vi "Make Necessary Directories.vi"(8 "error in":errorcluster, 11 "Path":path) -> (0 "error out":errorcluster, 3 "Duplicated path":path)   [LabVIEW 2013]
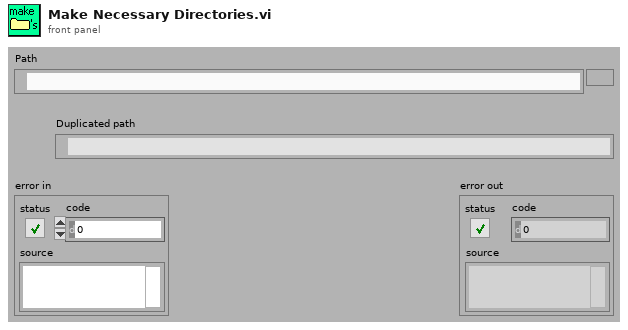
[diagram p1: front panel]
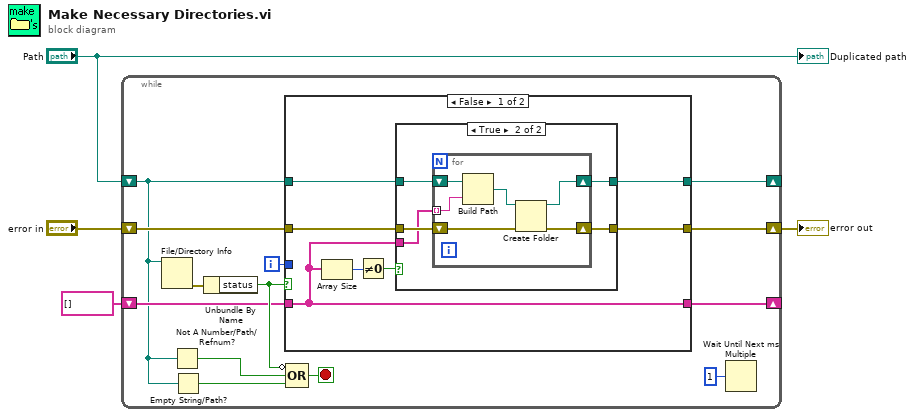
[diagram p0: block diagram]
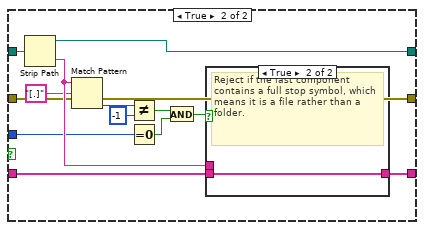
[diagram p3: hidden frame]
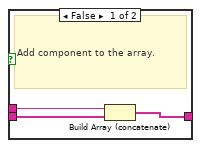
[diagram p4: hidden frame]
diagram:
  n1 = while {
    shift-right: [w14] -> _
    shift-left: "Path" -> [w8]
    shift-right: [w12] -> _
    shift-left: string[] [] -> [w13]
    shift-right: [w9] -> w1
    shift-left: "error in" -> [w10]
    i -> [w5]
    stop <- w16 stop-if-true
    n2 = File/Directory Info(path=w8) -> (error out=w17:errorcluster)  [unwired: 1 in, 6 out]
    n3 = Not A Number/Path/Refnum?(number/path/refnum=w8) -> (NaN/Path/Refnum?=w7:bool)
    n4 = Empty String/Path?(string/path=w8) -> (empty?=w6:bool)
    n5 = Unbundle By Name(w17) -> ("status"=w15:bool)
    n6 = case shown="False" w15 {
      tunnel: w8 -> [w24 w43]
      tunnel: [w23 w50] -> w14
      tunnel: w13 -> [w18 w49]
      tunnel: [w18 w48] -> w12
      tunnel: w10 -> [w22 w42]
      tunnel: [w19 w42] -> w9
      tunnel: w5 -> [_ w39]
      frame False {
        n7 = Array Size(array=w18) -> (size(s)=w20:i32)
        n8 = Not Equal To 0?(x=w20) -> (x != 0?=w21:bool)
        n9 = case shown="True" w21 {
          tunnel: w24 -> [w26 w31]
          tunnel: [w26 w29] -> w23
          tunnel: w22 -> [w25 w28]
          tunnel: w18 -> [_ w27]
          tunnel: [w25 w30] -> w19
          frame False {
          }
          frame True {
            n10 = for {
              shift-right: [w33] -> w29
              shift-left: w31 -> [w37]
              tunnel: w27 -> [w32] mode=indexing
              shift-right: [w34] -> w30
              shift-left: w28 -> [w35]
              n11 = Build Path(base path=w37, name or relative path=w32) -> (appended path=w36:path)
              n12 = Create Folder(path (use dialog)=w36, error in=w35) -> (created path=w33:path, error out=w34:errorcluster)  [unwired: 2 out]
            }
          }
        }
      }
      frame True {
        n13 = Strip Path(path=w43) -> (stripped path=w50:path, name=w47:string)
        n14 = Match Pattern(string=w47, regular expression="[.]") -> (offset past match=w46:i32)  [unwired: 4 out]
        n15 = Not Equal?(x=w46, y=-1) -> (x != y?=w41:bool)
        n16 = Equal To 0?(x=w39) -> (x = 0?=w38:bool)
        n17 = And(x=w41, y=w38) -> (x .and. y?=w40:bool)
        n18 = case shown="True" w40 {
          tunnel: w49 -> [w51 w54]
          tunnel: [w53 w54] -> w48
          tunnel: w47 -> [w52 _]
          frame False {
            # "Add component to the array."
            n19 = Build Array (concatenate)(w52, w51) -> (w53:string[])
          }
          frame True {
            # "Reject if the last component contains a full stop symbol, which means it is a file rather than a folder."
          }
        }
      }
    }
    n20 = Compound Arithmetic op=OR(invert w15, w7, w6) -> (w16:bool)
    n21 = Wait Until Next ms Multiple(millisecond multiple=u32 1) -> ()  [unwired: 1 out]
  }
  "error out" <- w1
  "Duplicated path" <- "Path"
